vi "Example Delaunay.vi"() -> ()   [LabVIEW 2023]
uses:
  <vilib>/numeric/Random Number (Range) DBL.vi
  LV QHull/QHull.lvlib
panel:
  out "size(s) 2":i32[](array[numeric])
  out "XY Graph":cluster{cluster{"number":dbl, "number":dbl}[]}[](graph)
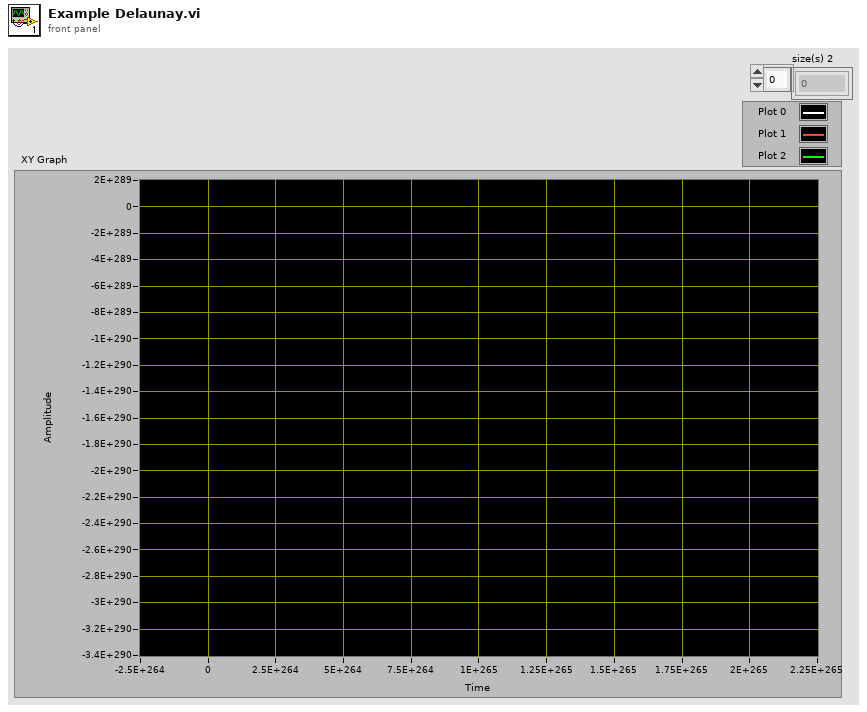
[diagram p1: front panel]
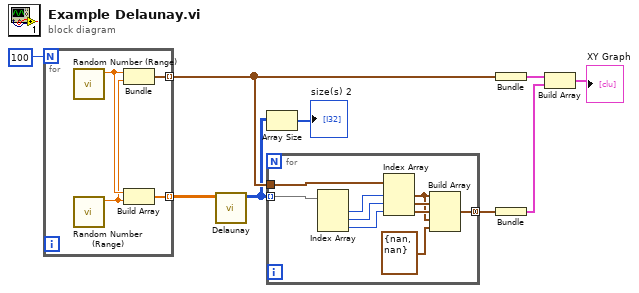
[diagram p0: block diagram]
diagram:
  n1 = for {
    N: 100 -> [_]
    tunnel: [w13] -> w9 mode=indexing
    tunnel: [w10] -> w4 mode=indexing
    n2 = call-poly <vilib>:"Random Number (Range).vi"() -> ("number"=w12:dbl)  [unwired: 11 in]
    n3 = call-poly <vilib>:"Random Number (Range).vi"() -> ("number"=w11:dbl)  [unwired: 11 in]
    n4 = Bundle("number"=w12, "number"=w11) -> (w10:cluster{"number":dbl, "number":dbl})  [unwired: 1 in]
    n5 = Build Array(w12, w11) -> (w13:dbl[])
  }
  n6 = call "Delaunay.vi"("points"=w9) -> ("simplices"=w2:i32[][])  [unwired: 9 in, 1 out]
  n7 = Array Size(array=w2) -> (size(s)=→"size(s) 2":i32[])
  n8 = for {
    tunnel: [w16] -> w3 mode=concatenating
    tunnel: w4 -> [w23]
    tunnel: w2 -> [w22] mode=indexing
    n9 = Index Array(array=w22) -> (element #1=w21:i32, element #2=w20:i32, element #3=w19:i32)  [unwired: 3 in]
    n10 = Index Array(array=w23, index #1=w21, index #2=w20, index #3=w19) -> (element #1=w15:cluster{"number":dbl, "number":dbl}, element #2=w18:cluster{"number":dbl, "number":dbl}, element #3=w17:cluster{"number":dbl, "number":dbl})
    n11 = Build Array(w15, w18, w17, w15, cluster{"number":dbl, "number":dbl} {"number"=nan, "number"=nan} ("element")) -> (w16:cluster{"number":dbl, "number":dbl}[])
  }
  n12 = Bundle(w4) -> (w7:cluster{cluster{"number":dbl, "number":dbl}[]})  [unwired: 1 in]
  n13 = Bundle(w3) -> (w5:cluster{cluster{"number":dbl, "number":dbl}[]})  [unwired: 1 in]
  n14 = Build Array(w7, w5) -> (→"XY Graph":cluster{cluster{"number":dbl, "number":dbl}[]}[])
